vi "takeHDRpic.vi"(8 "Frames to average":i32=1, 10 "Exposure Array":dbl[](array[numeric])) -> (2 "imgHDR":dbl[][](array[numeric]))   [LabVIEW 2016]
uses:
  <vilib>/Utility/error.llb/DialogType.ctl
panel:
  out "i":i32
  out "Show Exposure":dbl[](array[numeric])
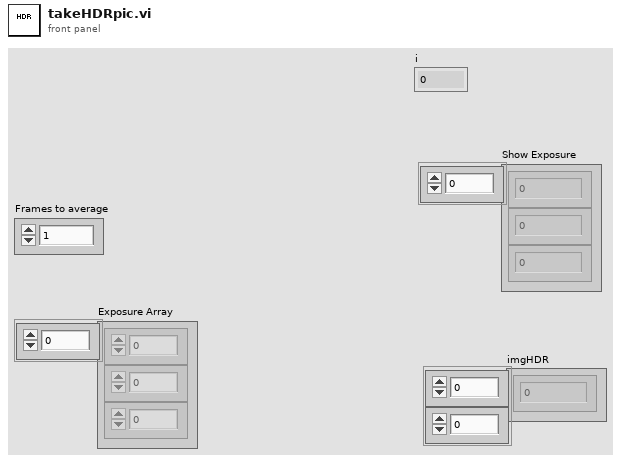
[diagram p1: front panel]
types:
  T1 = typedef "DialogType.ctl" = u16
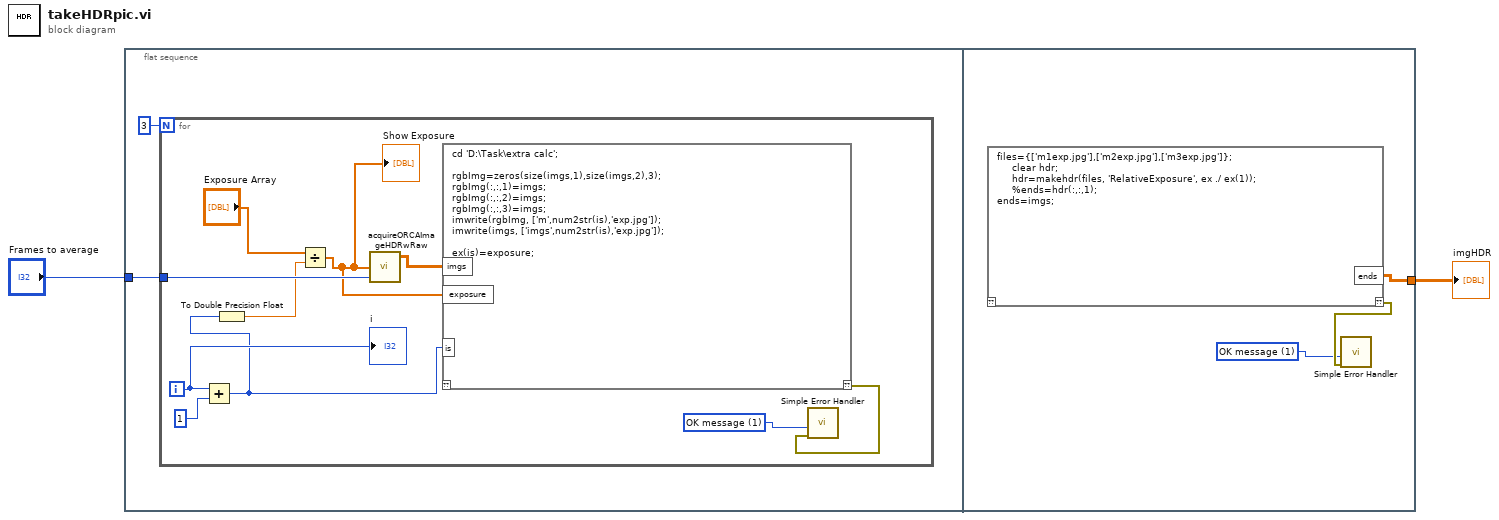
[diagram p0: block diagram]
diagram:
  n1 = flat-sequence {
    tunnel: "Frames to average" -> [w3]
    tunnel: [w17] -> w1
    frame #0 {
      n2 = for {
        N: 3 -> [_]
        tunnel: w3 -> [w14]
        i -> [w7]
        w11 = T1 1 items=["no dialog", "OK message", "continue or stop message", "OK message + warnings", "continue/stop + warnings"] ("type of dialog (OK msg:1)")
        n3 = Add(x=w7, y=1) -> (x+y=w6:i32)
        n4 = To Double Precision Float(number=w6) -> (double precision float=w13:dbl)
        n5 = Divide(x="Exposure Array", y=w13) -> (x/y=w8:dbl[])
        "Show Exposure" <- w8
        n6 = call "acquireORCAImageHDRwRaw.vi"("Average"=w14, "Exposure Array"=w8) -> ("imgHDR"=w5:dbl[][])  [unwired: 2 in, 1 out]
        n7 = script code="cd 'D:\\Task\\extra calc';\n\nrgbImg=zeros(size(imgs,1),size(imgs,2),3);\nrgbImg(:,:,1)=imgs;\nrgbImg(:,:,2)=imgs;\nrgbImg(:,:,3)=imgs;\nimwrite(rgbImg, ['m',num2str(is),'exp.jpg']);\nimwrite(imgs, ['imgs',num2str(is),'exp.jpg']);\n\nex(is)=exposure;"("imgs"=w5, "exposure"=w8, "is"=w6) -> ("??"=w12:errorcluster)  [unwired: 1 in]
        n8 = call <vilib>:"Simple Error Handler.vi"("type of dialog (OK msg:1)"=w11, "error in (no error)"=w12) -> ()  [unwired: 3 in, 5 out]
        "i" <- w7
      }
    }
    frame #1 {
      w15 = T1 1 items=["no dialog", "OK message", "continue or stop message", "OK message + warnings", "continue/stop + warnings"] ("type of dialog (OK msg:1)")
      n9 = script code="files={['m1exp.jpg'],['m2exp.jpg'],['m3exp.jpg']};\n     clear hdr;\n     hdr=makehdr(files, 'RelativeExposure', ex ./ ex(1));\n     %ends=hdr(:,:,1);\nends=imgs;"() -> ("??"=w16:errorcluster, "ends"=w17:dbl[][])  [unwired: 1 in]
      n10 = call <vilib>:"Simple Error Handler.vi"("type of dialog (OK msg:1)"=w15, "error in (no error)"=w16) -> ()  [unwired: 3 in, 5 out]
    }
  }
  "imgHDR" <- w1
